vi "Replicate.vi"(8 "error in (no error)":errorcluster, 9 "Direction Offset":i32, 10 "Current Position":T3, 11 "Test in":refnum<class "Swarm.lvclass">) -> (0 "error out":errorcluster, 1 "Direction":T1, 2 "Action":T2, 3 "Test out":refnum<class "Swarm.lvclass">, 4 "Replicated":refnum<class "Swarm.lvclass">)   [LabVIEW 2016, in "Swarm.lvclass"]
uses:
  Swarm.lvclass
  Common/Position.ctl
  Type Defs/Action Enum.ctl
  Type Defs/Direction Enum.ctl
  Swarm.lvclass/Swarm.ctl
  Type Defs/SB Type Defs.lvlib
  Common/Common.lvlib
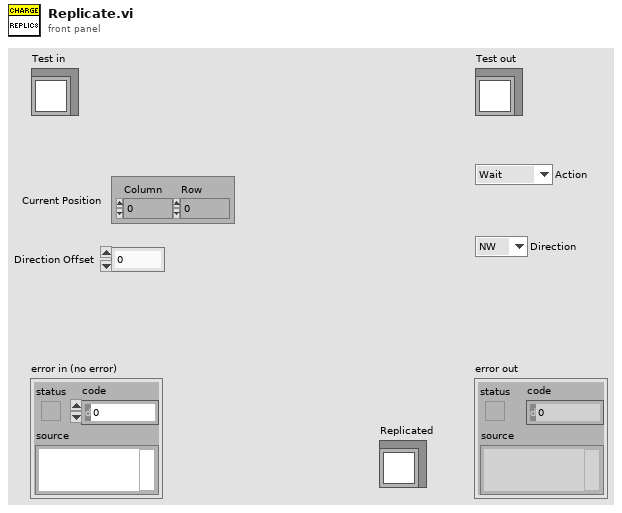
[diagram p1: front panel]
types:
  T1 = typedef "SB Type Defs.lvlib/Direction Enum.ctl" = enum16{"NW", "N", "NE", "E", "SE", "S", "SW", "W"}
  T2 = typedef "SB Type Defs.lvlib/Action Enum.ctl" = enum16{"Wait", "Move", "Attack", "Replicate"}
  T3 = typedef "Common.lvlib/Position.ctl" = cluster{"Column":i32, "Row":i32}
  T4 = typedef "Common.lvlib/Map DVR.ctl" = refnum<data-value>
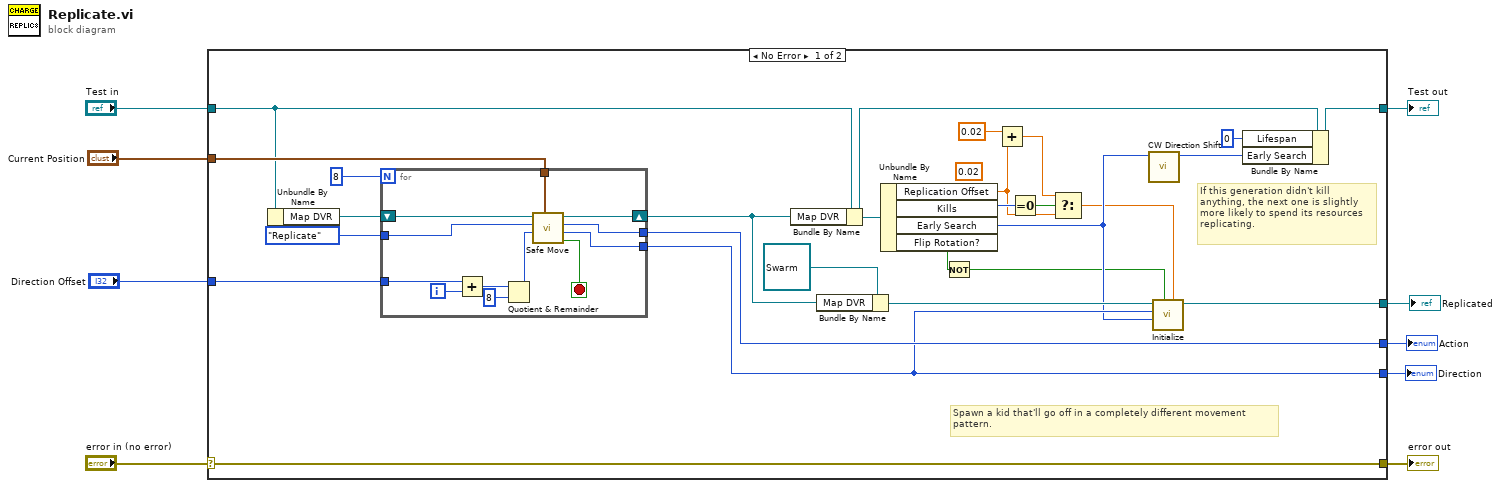
[diagram p0: block diagram]
diagram:
  n1 = case shown="No Error" "error in (no error)" {
    selector: "error in (no error)" -> [w35 w49]
    tunnel: [w35 w49] -> w8
    tunnel: [w21 w48] -> w6
    tunnel: "Test in" -> [w28 w48]
    tunnel: "Current Position" -> [w29 _]
    tunnel: [w24 _] -> w4
    tunnel: [w23 _] -> w3
    tunnel: [w27 _] -> w2
    tunnel: "Direction Offset" -> [w26 _]
    frame No Error {
      (unwired) 0.02 ("x")
      # "If this generation didn't kill\nanything, the next one is slightly\nmore likely to spend its resources\nreplicating."
      # "Spawn a kid that'll go off in a completely different movement\npattern."
      n2 = Unbundle By Name(w28) -> ("Map DVR"=w32:T4)
      n3 = for {
        N: 8 -> [_]
        tunnel: Action_Enum."Replicate" ("Desired Action") -> [w47]
        tunnel: w29 -> [w44]
        shift-right: [w45] -> w33
        shift-left: w32 -> [w46]
        tunnel: [w42] -> w27
        tunnel: [w41] -> w23
        tunnel: w26 -> [w36]
        i -> [w40]
        stop <- w43 stop-if-true
        n4 = Add(x=w36, y=w40) -> (x+y=w39:i32)
        n5 = Quotient & Remainder(x=w39, y=8) -> (x-y*floor(x/y)=w37:i32)  [unwired: 1 out]
        n6 = call "Safe Move.vi"("Position in"=w44, "Direction in"=w37, "Desired Action"=w47, "Map DVR"=w46) -> ("Accepted?"=w43:bool, "Direction"=w41:T1, "Action"=w42:T2, "Map DVR out"=w45:T4)  [unwired: 4 in]
      }
      n7 = Bundle By Name(cluster=w28, "Map DVR"=w33) -> (w22:refnum<class "Swarm.lvclass">)
      n8 = Bundle By Name(cluster=refnum<class "Swarm.lvclass"> refnum ("Test In"), "Map DVR"=w33) -> (w25:refnum<class "Swarm.lvclass">)
      n9 = Unbundle By Name(w22) -> ("Replication Offset"=w12:dbl, "Kills"=w13:i32, "Early Search"=w19:T1, "Flip Rotation?"=w17:bool)
      n10 = Not(x=w17) -> (.not. x?=w16:bool)
      n11 = Add(x=0.02, y=w12) -> (x+y=w15:dbl)
      n12 = Equal To 0?(x=w13) -> (x = 0?=w14:bool)
      n13 = Select(t=w15, s=w14, f=w12) -> (s? t:f=w11:dbl)
      n14 = call "CW Direction Shift.vi"("Direction"=w19) -> ("Numeric"=w18:i32)  [unwired: 10 in]
      n15 = call-dynamic "Initialize.vi"("Replication Offset"=w11, "Flip Rotation?"=w16, "Spawner Early Search"=w19, "Initial Direction Offset"=w23, "Test in"=w25) -> ("Test out"=w24:refnum<class "Swarm.lvclass">)  [unwired: 5 in, 1 out]
      n16 = Bundle By Name(cluster=w22, "Lifespan"=0, "Early Search"=w18) -> (w21:refnum<class "Swarm.lvclass">)
    }
    frame Error {
    }
  }
  "error out" <- w8
  "Test out" <- w6
  "Replicated" <- w4
  "Action" <- w2
  "Direction" <- w3
